vi "Build new run group.vi"(8 "error in (no error)":errorcluster, 9 "Numeric":i32, 10 "Run ID":i32, 11 "Daily datafile":T1 format="%.0x") -> (0 "error out":errorcluster, 3 "Daily datafile":T1 format="%.0x")   [LabVIEW 2016]
uses:
  <vilib>/addons/h5labview2/base/hid_t.ctl
  <vilib>/addons/h5labview2/base/lib_path.vi
  <vilib>/addons/h5labview2/base/H5Equery.vi
  Global Variables/GPS Position.vi
  <vilib>/addons/h5labview2/attrib/H5Awrite.llb/H5Awrite.xnode
  <vilib>/addons/h5labview2/group/H5G.lvlib
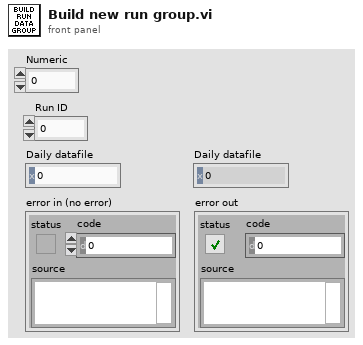
[diagram p1: front panel]
types:
  T1 = typedef "hid_t.ctl" = i32
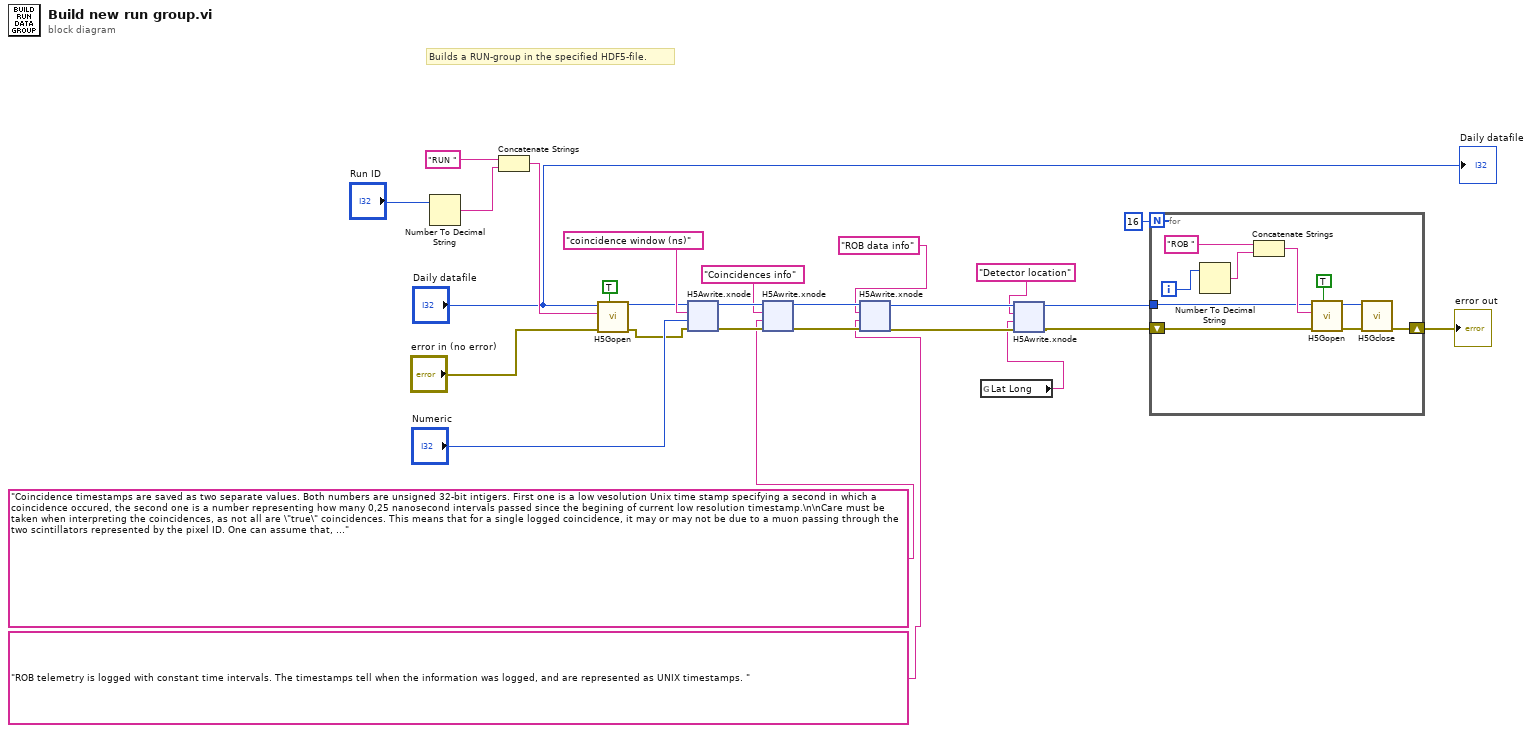
[diagram p0: block diagram]
diagram:
  # "Builds a RUN-group in the specified HDF5-file."
  n1 = Number To Decimal String(number="Run ID") -> (decimal integer string=w25:string)  [unwired: 1 in]
  n2 = Concatenate Strings("RUN " ("name"), w25) -> (w24:string)
  n3 = call <vilib>:"H5Gopen.vi"("create? (F)"=TRUE, "error in (no error)"="error in (no error)", "name"=w24, "ref in"="Daily datafile") -> ("error out"=w19:errorcluster, "group out"=w16:T1)  [unwired: 6 in]
  n4 = xnode "H5Awrite.xnode"("error in (no error)"=w19, "data"="Numeric", "attrib name"="coincidence window (ns)", "ref in"=w16) -> ("error out"=w15:errorcluster, "ref out"=w14:i32)  [unwired: 3 in, 1 out]
  n5 = xnode "H5Awrite.xnode"("error in (no error)"=w15, "data"="Coincidence timestamps are saved as two separate values. Both numbers are unsigned 32-bit intigers. First one is a low vesolution Unix time stamp specifying a second in which a coincidence occured, the second one is a number representing how many 0,25 nanosecond intervals passed since the begining of current low resolution timestamp.\n\nCare must be taken when interpreting the coincidences, as not all are \"true\" coincidences. This means that for a single logged coincidence, it may or may not be due to a muon passing through the two scintillators represented by the pixel ID. One can assume that, if there are no other coincidences in the same plane within +-15 nanoseconds, it is a true coincidence. If there are multiple coincidences closely spaced in time, some of them may be false. This ambiguity comes from the fact that two (or more) simultaneous muons may hit four (or more) different scintillators. If this happens, the four scintillators will each generate a signal, and the coincidence algorithm will be unable to distinguish whether it was four or two muons that impacted.  " ("object name"), "attrib name"="Coincidences info" ("object name"), "ref in"=w14) -> ("error out"=w12:errorcluster, "ref out"=w13:i32)  [unwired: 3 in, 1 out]
  n6 = xnode "H5Awrite.xnode"("error in (no error)"=w12, "data"="ROB telemetry is logged with constant time intervals. The timestamps tell when the information was logged, and are represented as UNIX timestamps. " ("object name"), "attrib name"="ROB data info" ("object name"), "ref in"=w13) -> ("error out"=w3:errorcluster, "ref out"=w6:i32)  [unwired: 3 in, 1 out]
  n7 = global read "GPS Position.vi" "Lat Long"() -> (w1:string)
  n8 = xnode "H5Awrite.xnode"("error in (no error)"=w3, "data"=w1, "attrib name"="Detector location" ("object name"), "ref in"=w6) -> ("error out"=w4:errorcluster, "ref out"=w5:i32)  [unwired: 3 in, 1 out]
  n9 = for {
    N: 16 -> [_]
    shift-right: [w30] -> w18
    shift-left: w4 -> [w37]
    tunnel: w5 -> [w31]
    i -> [w36]
    n10 = Number To Decimal String(number=w36) -> (decimal integer string=w35:string)  [unwired: 1 in]
    n11 = Concatenate Strings("ROB " ("name"), w35) -> (w33:string)
    n12 = call <vilib>:"H5Gopen.vi"("create? (F)"=TRUE, "error in (no error)"=w37, "name"=w33, "ref in"=w31) -> ("error out"=w28:errorcluster, "group out"=w29:T1)  [unwired: 6 in]
    n13 = call <vilib>:"H5Gclose.vi"("error in (no error)"=w28, "group in"=w29) -> ("error out"=w30:errorcluster)  [unwired: 9 in]
  }
  "error out" <- w18
  "Daily datafile" <- "Daily datafile"
